vi "Set Temperature Coefficient.vi"(0 "EPU452 in":refnum<class "EPU452.lvclass">, 5 "Channel":T1, 7 "Temperature Coefficient (%/°C)":dbl, 9 "Reference(°C)":dbl, 11 "error in (no error)":errorcluster) -> (4 "EPU452 out":refnum<class "EPU452.lvclass">, 15 "error out":errorcluster)   [LabVIEW 2018, in "EPU452.lvclass"]
uses:
  EPU452.lvclass
  Controls/Channels.ctl
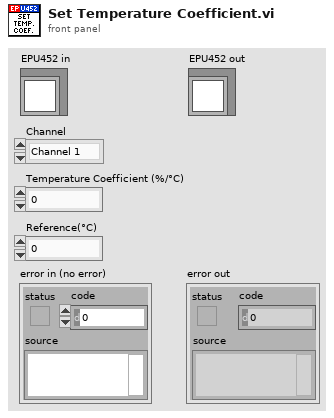
[diagram p1: front panel]
types:
  T1 = typedef "EPU452.lvclass/Channels.ctl" = enum16{"Channel 1", "Channel 2", "Channel 3", "Channel 4"}
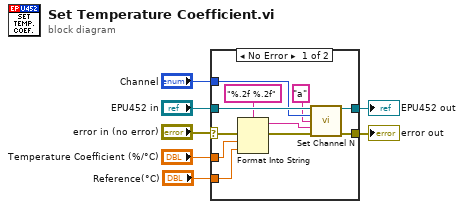
[diagram p0: block diagram]
diagram:
  n1 = case shown="No Error" "error in (no error)" {
    selector: "error in (no error)" -> [w13 w20]
    tunnel: [w16 w20] -> w6
    tunnel: [w17 w19] -> w4
    tunnel: "EPU452 in" -> [w18 w19]
    tunnel: "Channel" -> [w15 _]
    tunnel: "Temperature Coefficient (%/°C)" -> [w10 _]
    tunnel: "Reference(°C)" -> [w8 _]
    frame No Error {
      n2 = Format Into String(format string="%.2f %.2f", error in=w13, w10, w8) -> (resulting string=w11:string, error out=w12:errorcluster)  [unwired: 1 in]
      n3 = call "Set Channel N.vi"("EPU452 in"=w18, "Channel"=w15, "Function"="a", "Argument/s"=w11, "error in (no error)"=w12) -> ("EPU452 out"=w17:refnum<class "EPU452.lvclass">, "error out"=w16:errorcluster)  [unwired: 8 in, 1 out]
    }
    frame Error {
    }
  }
  "error out" <- w6
  "EPU452 out" <- w4
